vi "Simple Solar Tracker v4.vi"() -> ()   [LabVIEW 2024]
uses:
  <vilib>/Instr/_visa.llb/VISA Configure Serial Port (Instr).vi
panel:
  in  "stop":bool
  out "Waveform Chart":dbl(graph)=129.23
  in  "Steps":dbl(slide)=11.224489795918368 scale=0.0..50.0
  out "Old":dbl=129.23
  out "New":dbl=129.23
  in  "Baud Rate  2":u32=115200
  in  "VISA resource":refnum<visa-resource-name>="COM56"
  in  "Delay":dbl(slide)=116.3265306122449 scale=100.0..200.0
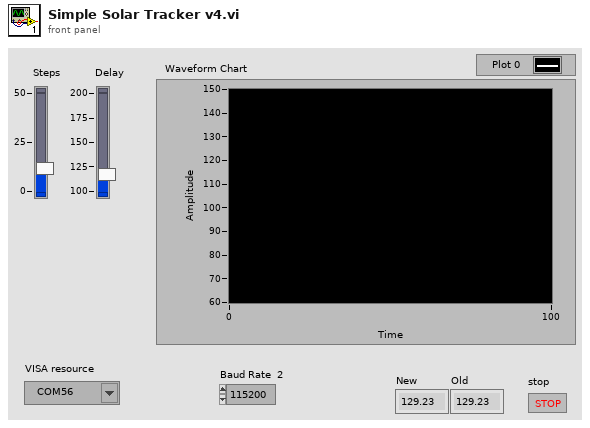
[diagram p1: front panel]
types:
  T1 = enum16{"init", "getVal", "Move", "quit", "setDir"}
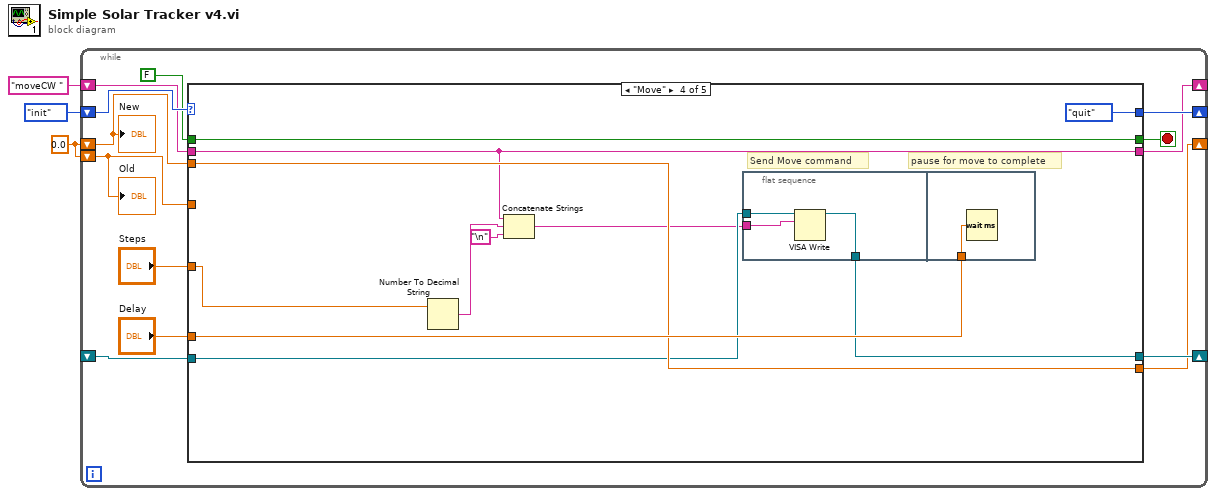
[diagram p0: block diagram]
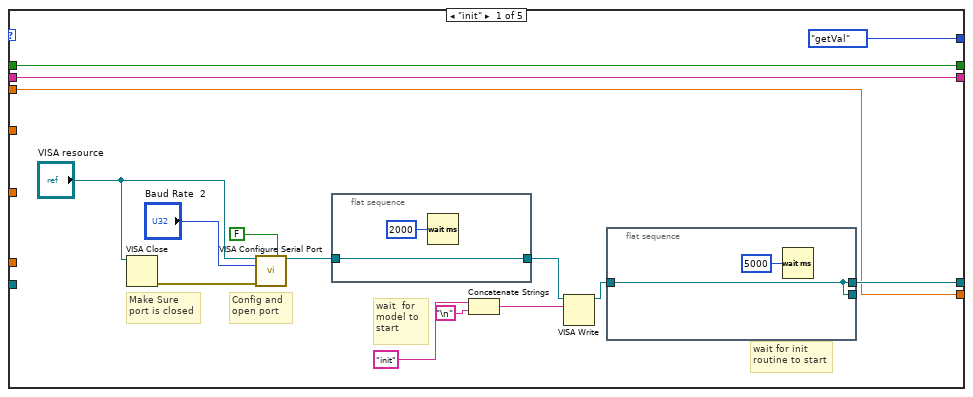
[diagram p2: hidden frame]
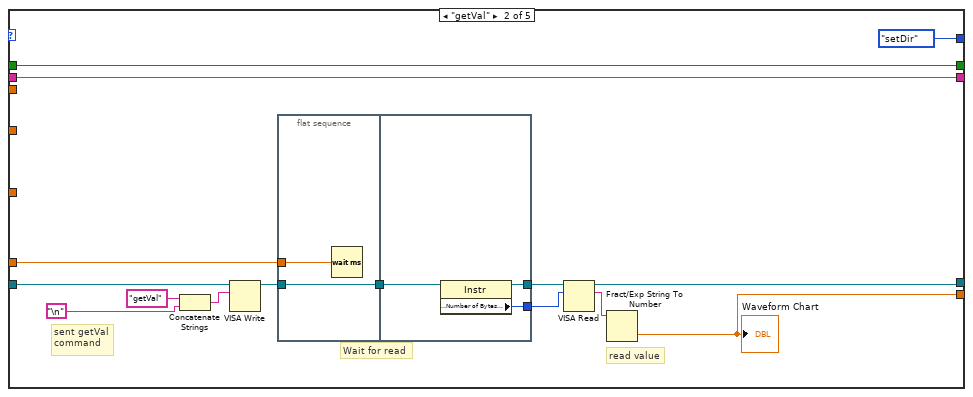
[diagram p3: hidden frame]
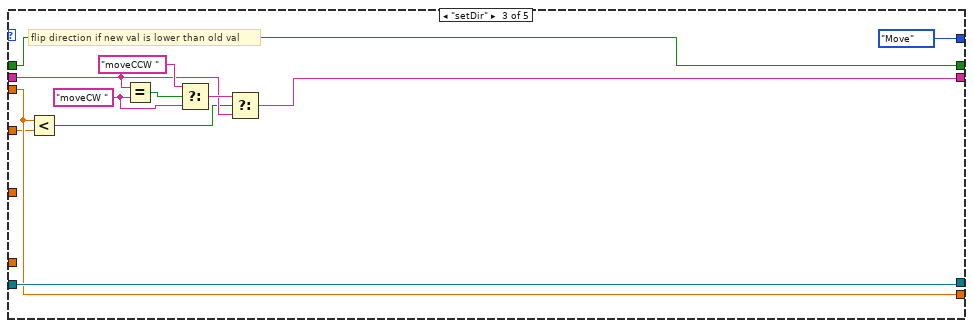
[diagram p4: hidden frame]
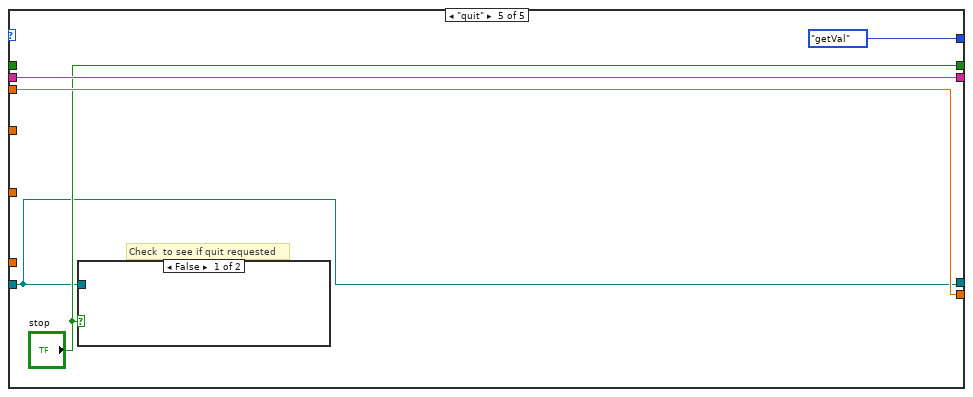
[diagram p5: hidden frame]
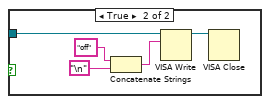
[diagram p6: hidden frame]
diagram:
  w1 = 0.0
  n1 = while {
    shift-right: [w16] -> _
    shift-left: T1."init" -> [w15]
    shift-right: [w14] -> _
    shift-left: _ -> [w13]
    shift-right: [w9] -> _
    shift-left: "moveCW " ("string") -> [w12]
    shift-right: [w10] -> _
    shift-left: w1 -> [w6]
    shift-left: w1 -> [w7]
    stop <- w5 stop-if-true
    n2 = case shown="\"Move\"" w15 {
      tunnel: [T1."getVal" T1."setDir" T1."Move" T1."quit" T1."getVal"] -> w16
      tunnel: [w21 w36 w63 w73 w83] -> w14
      tunnel: w13 -> [_ w46 w63 w75 w83]
      tunnel: w12 -> [w19 w42 w60 w70 w87]
      tunnel: "Delay" -> [_ w43 _ w78 _]
      tunnel: [w20 w41 w59 w77 w86] -> w10
      tunnel: w6 -> [w20 _ w59 w77 w86]
      tunnel: w7 -> [_ _ w58 _ _]
      tunnel: [w19 w42 w56 w70 w87] -> w9
      tunnel: "Steps" -> [_ _ _ w71 _]
      tunnel: [w18 w40 w62 w76 "stop"] -> w5
      tunnel: FALSE -> [w18 w40 w62 w76 _]
      frame "init" {
        # "wait for init\nroutine to start"
        # "wait  for\nmodel to \nstart"
        # "Config and\nopen port"
        # "Make Sure\nport is closed"
        n3 = VISA Close(VISA resource name="VISA resource") -> (error out=w29:errorcluster)  [unwired: 1 in]
        n4 = call-poly "VISA Configure Serial Port"("VISA resource name"="VISA resource", "Enable Termination\nChar (T)"=FALSE ("Enable Termination\nChar (T)"), "baud rate (9600)"="Baud Rate  2", "error in (no error)"=w29) -> ("VISA resource name out"=w30:refnum<visa-resource-name>)  [unwired: 10 in, 1 out]
        n5 = flat-sequence {
          tunnel: w30 -> [w34]
          tunnel: [w34] -> w22
          frame #0 {
            n6 = Wait (ms)(milliseconds to wait=u32 2000) -> ()  [unwired: 1 out]
          }
        }
        n7 = Concatenate Strings("init" ("string"), "\n") -> (w25:string)
        n8 = VISA Write(VISA resource name=w22, write buffer=w25) -> (VISA resource name out=w23:refnum<visa-resource-name>)  [unwired: 1 in, 2 out]
        n9 = flat-sequence {
          tunnel: w23 -> [w32]
          tunnel: [w32] -> _
          tunnel: [w32] -> w21
          frame #0 {
            n10 = Wait (ms)(milliseconds to wait=u32 5000) -> ()  [unwired: 1 out]
          }
        }
      }
      frame "getVal" {
        # "read value"
        # "Wait for read"
        # "sent getVal\ncommand"
        n11 = Concatenate Strings("getVal" ("string"), "\n") -> (w48:string)
        n12 = VISA Write(VISA resource name=w46, write buffer=w48) -> (VISA resource name out=w37:refnum<visa-resource-name>)  [unwired: 1 in, 2 out]
        n13 = flat-sequence {
          tunnel: w43 -> [w52]
          tunnel: w37 -> [w51]
          tunnel: [w51] -> w38
          tunnel: [w55] -> w45
          tunnel: [w54] -> w39
          tunnel: w38 -> [w53]
          frame #0 {
            n14 = Wait (ms)(milliseconds to wait=w52) -> ()  [unwired: 1 out]
          }
          frame #1 {
            n15 = property class="Instr"(reference=w53) -> (reference out=w55:refnum<visa-resource-name>, "Serial Settings:Number of Bytes at Serial Port"=w54:u32)  [unwired: 1 in, 1 out]
          }
        }
        n16 = VISA Read(VISA resource name=w45, byte count=w39) -> (VISA resource name out=w36:refnum<visa-resource-name>, read buffer=w44:string)  [unwired: 1 in, 2 out]
        n17 = Fract/Exp String To Number(string=w44) -> (number=w41:dbl)  [unwired: 3 in, 1 out]
        "Waveform Chart" <- w41
      }
      frame "setDir" {
        w66 = "moveCW " ("string")
        # "flip direction if new val is lower than old val"
        n18 = Less?(x=w59, y=w58) -> (x < y?=w57:bool)
        n19 = Equal?(x=w60, y=w66) -> (x = y?=w67:bool)
        n20 = Select(t="moveCCW " ("string"), s=w67, f=w66) -> (s? t:f=w64:string)
        n21 = Select(t=w64, s=w57, f=w60) -> (s? t:f=w56:string)
      }
      frame "Move" {
        # "pause for move to complete"
        # "Send Move command"
        n22 = Number To Decimal String(number=w71) -> (decimal integer string=w69:string)  [unwired: 1 in]
        n23 = Concatenate Strings(w70, w69, "\n") -> (w68:string)
        n24 = flat-sequence {
          tunnel: w75 -> [w80]
          tunnel: w68 -> [w81]
          tunnel: [w79] -> w73
          tunnel: w78 -> [w82]
          frame #0 {
            n25 = VISA Write(VISA resource name=w80, write buffer=w81) -> (VISA resource name out=w79:refnum<visa-resource-name>)  [unwired: 1 in, 2 out]
          }
          frame #1 {
            n26 = Wait (ms)(milliseconds to wait=w82) -> ()  [unwired: 1 out]
          }
        }
      }
      frame "quit" {
        # "Check  to see if quit requested"
        n27 = case shown="False" "stop" {
          tunnel: w83 -> [_ w88]
          frame False {
          }
          frame True {
            n28 = Concatenate Strings("off" ("string"), "\n") -> (w91:string)
            n29 = VISA Write(VISA resource name=w88, write buffer=w91) -> (VISA resource name out=w92:refnum<visa-resource-name>)  [unwired: 1 in, 2 out]
            n30 = VISA Close(VISA resource name=w92) -> ()  [unwired: 1 in, 1 out]
          }
        }
      }
    }
    "Old" <- w7
    "New" <- w6
  }
